vi "State Controller Test.vi"() -> ()   [LabVIEW 2016]
panel:
  in  "Start":bool
  in  "stop":bool
  out "Current State":string
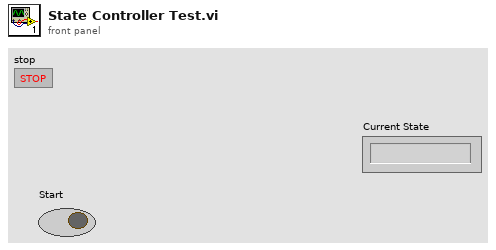
[diagram p1: front panel]
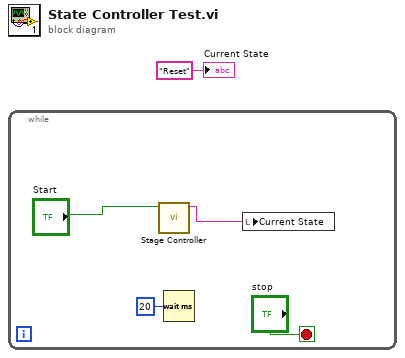
[diagram p0: block diagram]
diagram:
  n1 = while {
    stop <- "stop" stop-if-true
    n2 = call "Stage Controller.vi"("Start!"="Start") -> ("Current State"=w3:string)  [unwired: 9 in, 1 out]
    n3 = Wait (ms)(milliseconds to wait=u32 20) -> ()  [unwired: 1 out]
    n4 = local write "Current State"(w3) -> ()
  }
  "Current State" <- "Reset" ("Current State")
